vi "Two Bytes to Number.vi"(0 "VISA resource name":refnum<visa-resource-name>, 2 "Input Command Frame":string, 5 "Index 0 (3)":i8=3 min=3 max=25, 7 "Index 1 (4)":i8=4 min=3 max=25, 11 "error in (no error)":errorcluster) -> (4 "VISA resource name out":refnum<visa-resource-name>, 8 "Numerical Value":dbl format="%#.3g", 15 "error out":errorcluster)   [LabVIEW 2019, in "BK Precision 178XB Series.lvlib"]
doc: "This VI scans through Input command frame string and takes two bytes out of the string selected by index 0 and index 1. Then, the bytes get arranged in little-endian format, converted from hexadecimal to integer, and formatted to a decimal value at the <b>Numerical Value</b> output."
uses:
  BK Precision 178XB Series.lvlib
panel:
  # "(c) 2009 B&K PRECISION CORPORATION.  ALL RIGHTS RESERVED."
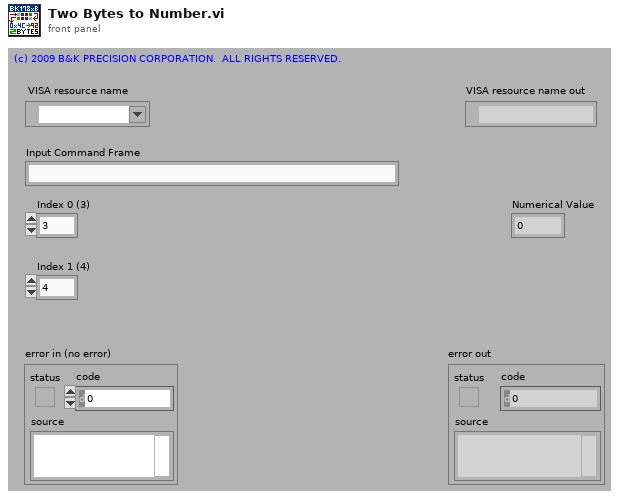
[diagram p1: front panel]
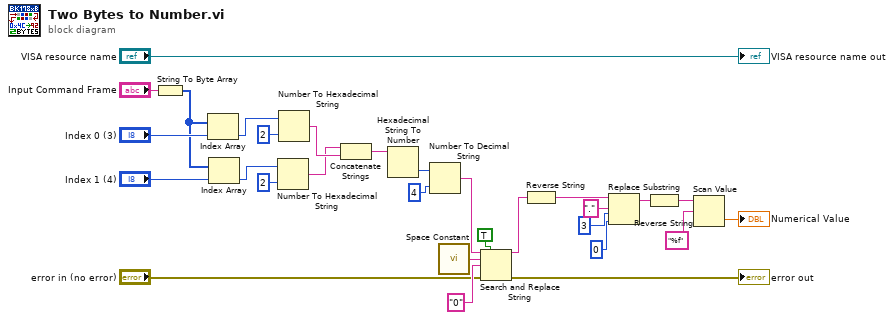
[diagram p0: block diagram]
diagram:
  n1 = String To Byte Array(string="Input Command Frame") -> (unsigned byte array=w26:u8[])
  n2 = Index Array(array=w26, index="Index 0 (3)") -> (element=w24:u8)
  n3 = Index Array(array=w26, index="Index 1 (4)") -> (element=w23:u8)
  n4 = Number To Hexadecimal String(1:2, 2:w23) -> (0:w21:string)
  n5 = Number To Hexadecimal String(1:2, 2:w24) -> (0:w22:string)
  n6 = Concatenate Strings(w21, w22) -> (w13:string)
  n7 = Hexadecimal String To Number(string=w13) -> (number=w6:u32)  [unwired: 2 in, 1 out]
  n8 = Number To Decimal String(number=w6, width (-)=4) -> (decimal integer string=w5:string)
  n9 = call <vilib>:"Space Constant.vi"() -> ("String"=w12:string)
  n10 = Search and Replace String(replace all?=TRUE, input string=w5, search string=w12, replace string="0", error in="error in (no error)") -> (result string=w4:string, error out=→"error out":errorcluster)  [unwired: 3 in, 2 out]
  n11 = Reverse String(1:w4) -> (0:w3:string)
  n12 = Replace Substring(2:0 ("length (len. of substring)"), 3:3 ("offset (0)"), 4:"." ("substring (\"\")"), 5:w3) -> (1:w2:string)  [unwired: 1 out]
  n13 = Reverse String(1:w2) -> (0:w14:string)
  n14 = Scan Value(string=w14, format string="%f") -> (value=→"Numerical Value":dbl)  [unwired: 1 in, 1 out]
  "VISA resource name out" <- "VISA resource name"
